vi "Init Module.vi"(8 "error in (no error)":errorcluster, 11 "Singleton Module Admin in":refnum<class "Delacor_lib_QMH_Module Admin.lvclass">) -> (0 "error out":errorcluster, 2 "Anode Request Events":T1, 3 "Singleton Module Admin out":refnum<class "Delacor_lib_QMH_Module Admin.lvclass">)   [LabVIEW 2024, in "Anode.lvlib"]
doc: "Initialize the module by creating Broadcast Events, Request Events, and synchronization rendezvous.\n_____\nBased on Delacor QMH Project Template 3.1.0.34.\n\n<b>Note:</b> This VI was modified by the <b>Validate DQMH Module</b> tool to add the 'Show Main VI Diagram on Init' functionality included in DQMH 6.1."
uses:
  Anode.lvlib
  <vilib>/Delacor/Delacor QMH/Libraries/Module Admin_class/Delacor_lib_QMH_Module Admin.lvclass
  Request Events--cluster.ctl
  Stop Argument--cluster.ctl
  Show Panel Argument--cluster.ctl
  Hide Panel Argument--cluster.ctl
  Get Module Execution Status Argument--cluster.ctl
  Show Diagram Argument--cluster.ctl
  Change Panel Argument--cluster.ctl
  <vilib>/MGI/Panel Manager/Panel/Panel/Panel.lvclass
  Set Anode Inlet Pressure SP Argument--cluster.ctl
  Initialise Pressure Regulator Interface Argument--cluster.ctl
  Modbus Config--cluster.ctl
  Start Polling Pressure Regulator Status Argument--cluster.ctl
  Stop Polling Pressure Regulator Status Argument--cluster.ctl
  Read Pressure Regulator Status Argument--cluster.ctl
  Set Pressure Regulator Control Function Argument--cluster.ctl
  Modbus Flexi-Flow API/Control Function Values--enum.ctl
  Set Anode Inlet Flow SP Argument--cluster.ctl
  Set Anode Inlet Valve State Argument--cluster.ctl
  Anode Solenoid Valve--enum.ctl
  Wake Connection Helper Loop Argument--cluster.ctl
  Set Anode Gas Supply Valve Argument--cluster.ctl
  Set Purge Valve Argument--cluster.ctl
  Set Purge Strategy Argument--cluster.ctl
  Purge Strategy--cluster.ctl
  Purge Strategy--enum.ctl
  Wake Purge Strategy Helper Loop Argument--cluster.ctl
  Update Purge Strategy Settings Argument--cluster.ctl
  Wake Purge Helper Loop Argument--cluster.ctl
  Wake Recirculation Pump Helper Loop Argument--cluster.ctl
  Sleep Recirculation Pump Helper Loop Argument--cluster.ctl
  Set Pump Speed SP Argument--cluster.ctl
  Set Pump Enable State Argument--cluster.ctl
  Set Pump Speed Control Mode Argument--cluster.ctl
  Update Purge Strategy Helper Loop Argument--cluster.ctl
  Force Purge Argument--cluster.ctl
  Reset Counter Argument--cluster.ctl
  Wake H2 Sensor Loop Argument--cluster.ctl
  Sleep H2 Sensor Loop Argument--cluster.ctl
  Start H2 Sensor Measurement Argument--cluster.ctl
  Stop H2 Sensor Measurement Argument--cluster.ctl
  Modbus Flexi-Flow API/Bronkhorst Flexi-Flow ModbusTCP API.lvlib
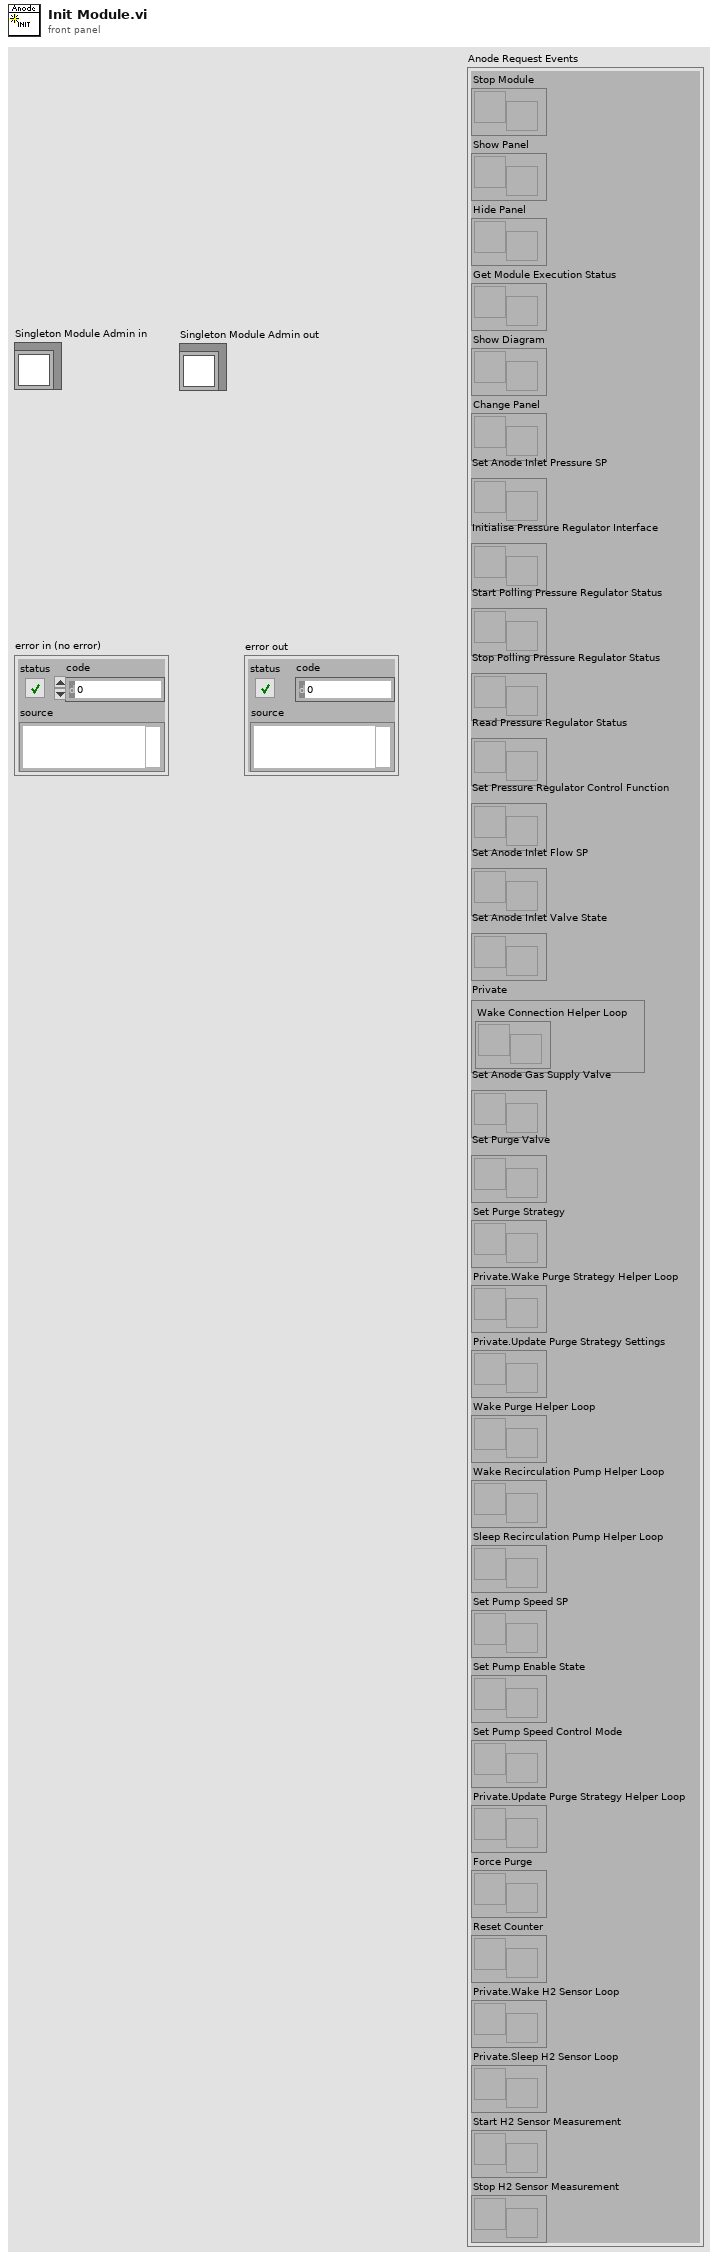
[diagram p1: front panel]
types:
  T1 = typedef "Anode.lvlib/Request Events--cluster.ctl" = cluster{"Stop Module":refnum<user-event>, "Show Panel":refnum<user-event>, "Hide Panel":refnum<user-event>, "Get Module Execution Status":refnum<user-event>, "Show Diagram":refnum<user-event>, "Change Panel":refnum<user-event>, "Set Anode Inlet Pressure SP":refnum<user-event>, "Initialise Pressure Regulator Interface":refnum<user-event>, "Start Polling Pressure Regulator Status":refnum<user-event>, "Stop Polling Pressure Regulator Status":refnum<user-event>, "Read Pressure Regulator Status":refnum<user-event>, "Set Pressure Regulator Control Function":refnum<user-event>, "Set Anode Inlet Flow SP":refnum<user-event>, "Set Anode Inlet Valve State":refnum<user-event>, "Private":cluster{"Wake Connection Helper Loop":refnum<user-event>}, "Set Anode Gas Supply Valve":refnum<user-event>, "Set Purge Valve":refnum<user-event>, "Set Purge Strategy":refnum<user-event>, "Private.Wake Purge Strategy Helper Loop":refnum<user-event>, "Private.Update Purge Strategy Settings":refnum<user-event>, "Wake Purge Helper Loop":refnum<user-event>, "Wake Recirculation Pump Helper Loop":refnum<user-event>, "Sleep Recirculation Pump Helper Loop":refnum<user-event>, "Set Pump Speed SP":refnum<user-event>, "Set Pump Enable State":refnum<user-event>, "Set Pump Speed Control Mode":refnum<user-event>, "Private.Update Purge Strategy Helper Loop":refnum<user-event>, "Force Purge":refnum<user-event>, "Reset Counter":refnum<user-event>, "Private.Wake H2 Sensor Loop":refnum<user-event>, "Private.Sleep H2 Sensor Loop":refnum<user-event>, "Start H2 Sensor Measurement":refnum<user-event>, "Stop H2 Sensor Measurement":refnum<user-event>}
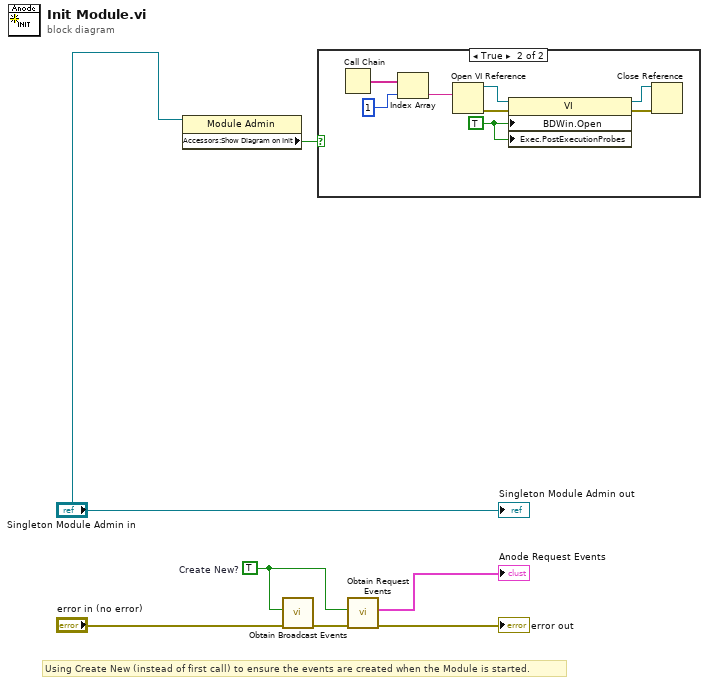
[diagram p0: block diagram]
diagram:
  w4 = TRUE  # Create New?
  # "Using Create New (instead of first call) to ensure the events are created when the Module is started."
  n1 = property class="Module Admin"(reference="Singleton Module Admin in") -> ("Accessors:Show Diagram on Init"=w1:bool)  [unwired: 1 in, 2 out]
  n2 = call "Obtain Broadcast Events.vi"("error in (no error)"="error in (no error)", "Create New?"=w4) -> ("error out"=w7:errorcluster)  [unwired: 8 in, 1 out]
  n3 = case shown="True" w1 {
    frame False {
    }
    frame True {
      w11 = TRUE ("Block Diagram Window:Open")
      n4 = Call Chain() -> (call chain=w15:string[])
      n5 = Index Array(array=w15, index=1) -> (element=w8:string)
      n6 = Open VI Reference(vi path=w8) -> (vi reference=w12:refnum<vi>, error out=w13:errorcluster)  [unwired: 5 in]
      n7 = property class="VI"(reference=w12, error in=w13, "BDWin.Open"=w11, "Exec.PostExecutionProbes"=w11) -> (reference out=w9:refnum<vi>, error out=w10:errorcluster)
      n8 = Close Reference(reference=w9, error in (no error)=w10) -> ()  [unwired: 1 out]
    }
  }
  n9 = call "Obtain Request Events.vi"("error in (no error)"=w7, "Create New?"=w4) -> ("error out"=→"error out":errorcluster, "Anode Request Events"=→"Anode Request Events":T1)  [unwired: 8 in]
  "Singleton Module Admin out" <- "Singleton Module Admin in"
